vi "Teleop.vi"(10 "Match Info":T1={"Autonomous Elapsed Seconds"=0.0, "TeleOp Elapsed Seconds"=0.0, "Disabled Elapsed Seconds"=0.0, "Visited Autonomous"=FALSE, "Visited TeleOp"=FALSE, "Visited Disabled"=FALSE, "Autonomous Settings"={"Autonomous Style"=enum."Independent", "VI Refnum"=refnum}}, 11 "Call Context":T2) -> ()   [LabVIEW 2015]
doc: "This VI is called for each TeleOp packet received from the DS where the robot is not disabled. It is often used to read from the joysticks and update I/O or to update setpoints for timed control loops. It should complete and return within 20 milliseconds or it may miss DS packets."
uses:
  <vilib>/Rock Robotics/WPI/DriverStation/WPI_DriverStationDerivedRobotMode.ctl
  <vilib>/Rock Robotics/WPI/DriverStation/WPI_DriverStationMatch Info.ctl
  <vilib>/Rock Robotics/WPI/CAN/TalonSRX/WPI_CANTalonSRX_APIControlMode.ctl
  Global Variables/Temp Variables.vi
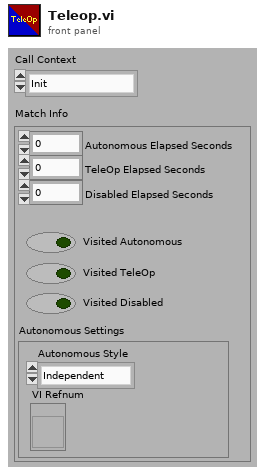
[diagram p1: front panel]
types:
  T1 = typedef "WPI_DriverStationMatch Info.ctl" = cluster{"Autonomous Elapsed Seconds":dbl, "TeleOp Elapsed Seconds":dbl, "Disabled Elapsed Seconds":dbl, "Visited Autonomous":bool, "Visited TeleOp":bool, "Visited Disabled":bool, "Autonomous Settings":cluster{"Autonomous Style":enum16{"Iterative", "Independent"}, "VI Refnum":refnum<vi>}}
  T2 = typedef "WPI_DriverStationDerivedRobotMode.ctl" = enum16{"Init", "Execute", "Stop"}
  T3 = typedef "WPI_CANTalonSRX_APIControlMode.ctl" = enum8{"Percent VBus", "Speed", "Position", "Slave", "Unchanged / Invalid", "Voltage Compensation", "Current", "Motion Profile"}
  T4 = typedef "Robot Control Outputs 2016.ctl" = cluster{"Pilot Left Joystick left-right":dbl, "Pilot Left Joystick up-down":dbl, "Pilot A Button":bool, "Pilot B Button":bool, "Pilot X Button":bool, "Pilot Y Button":bool, "Pilot Left Bumper":bool, "Pilot Right Bumper":bool, "Pilot Back Button":bool, "Pilot Start Button":bool, "Pilot Left Joystick Press":bool, "Pilot Right Joystick Press":bool, "Pilot Left Trigger":dbl, "Pilot Right Joystick left-right":dbl, "Pilot Right Joystick up-down":dbl, "Pilot Right Trigger":dbl, "Copilot Left Joystick left-right":dbl, "Copilot Left Joystick up-down":dbl, "Copilot A Button":bool, "Copilot B Button":bool, "Copilot X Button":bool, "Copilot Y Button":bool, "Copilot Left Bumper":bool, "Copilot Right Bumper":bool, "Copilot Back Button":bool, "Copilot Start Button":bool, "Copilot Left Joystick Press":bool, "Copilot Right Joystick Press":bool, "Copilot Left Trigger":dbl, "Copilot Right Joystick left-right":dbl, "Copilot Right Joystick up-down":dbl, "Copilot Right Trigger":dbl}
  T5 = typedef "Robot Commands 2016.ctl" = cluster{"Robot Forward-Back":dbl, "Robot Twist":dbl, "Fire":bool, "Lift/Drive Shift":bool, "Raise Lifter":bool, "Raise Grabber":bool, "Lower Grabber":bool, "Roller":T6, "Robot Climb Both Sides":dbl, "Grabber to Middle Position":bool, "Grabber to Top Position":bool, "Grabber to Bottom Position":bool, "Robot Climb Left Side":dbl, "Robot Climb Right Side":dbl, "Speed Control Left Side":dbl, "Speed Control Right Side":dbl, "Lower Lifter":bool, "Defense Mode":bool, "Deploy Lifter":bool, "Auto Targetting":bool, "Do the Jiggle":bool}
  T6 = typedef "Roller State.ctl" = enum16{"DONT MOVE", "Intake", "Outtake"}
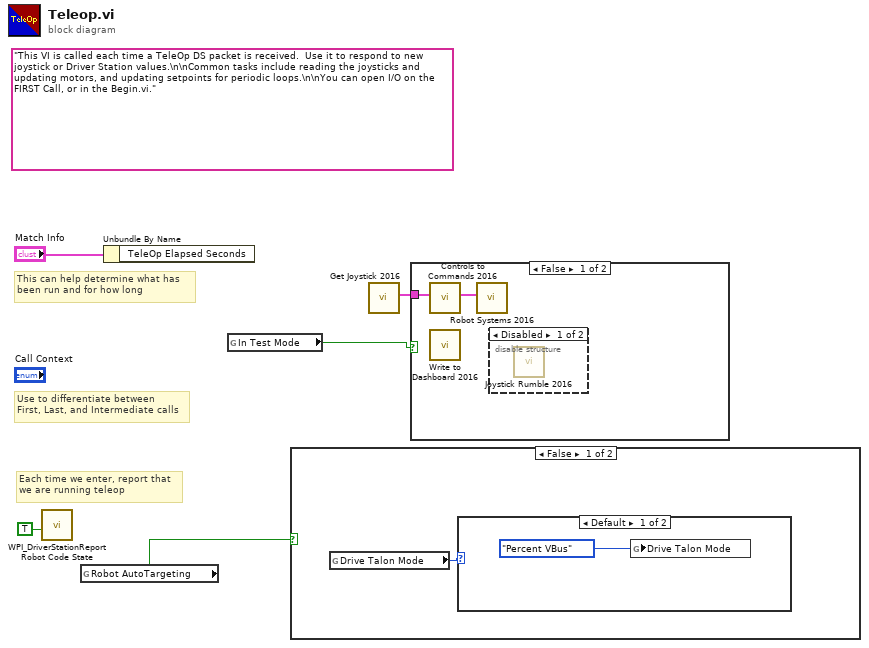
[diagram p0: block diagram]
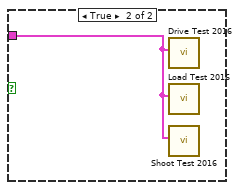
[diagram p5: hidden frame]
diagram:
  (unwired) "This VI is called each time a TeleOp DS packet is received.  Use it to respond to new joystick or Driver Station values.\n\nCommon tasks include reading the joysticks and updating motors, and updating setpoints for periodic loops.\n\nYou can open I/O on the FIRST Call, or in the Begin.vi."
  # "Each time we enter, report that\nwe are running teleop"
  # "Use to differentiate between\nFirst, Last, and Intermediate calls"
  # "This can help determine what has\nbeen run and for how long"
  n1 = call <vilib>:"WPI_DriverStationReport Robot Code State.vi"("TeleOp"=TRUE ("Autonomous")) -> ()  [unwired: 10 in, 1 out]
  n2 = global read "Temp Variables.vi" "Robot AutoTargeting"() -> (w1:bool)
  n3 = Unbundle By Name("Match Info") -> ()  [unwired: 1 out]
  n4 = global read "Temp Variables.vi" "In Test Mode"() -> (w2:bool)
  n5 = case shown="False" w1 {
    frame False {
      n6 = global read "Temp Variables.vi" "Drive Talon Mode"() -> (w6:T3)
      n7 = case shown="Default" w6 {
        frame Default {
          n8 = global write "Temp Variables.vi" "Drive Talon Mode"(WPI_CANTalonSRX_APIControlMode."Percent VBus" ("Drive Talon Mode")) -> ()
        }
        frame "Percent VBus" {
        }
      }
    }
    frame True {
    }
  }
  n9 = call "Get Joystick 2016.vi"() -> ("Pilot-CoPilot Controls"=w3:T4)  [unwired: 11 in]
  n10 = case shown="False" w2 {
    tunnel: w3 -> [w9 w10]
    frame False {
      n11 = call "Controls to Commands 2016.vi"("Pilot-CoPilot Controls"=w9) -> ("Robot Commands"=w8:T5)  [unwired: 10 in]
      n12 = call "Write to Dashboard 2016.vi"() -> ()  [unwired: 12 in]
      n13 = call "Robot Systems 2016.vi"("Robot Commands"=w8) -> ()  [unwired: 11 in]
      n14 = disable-structure shown="Disabled" {
        frame Disabled {
          n15 = call "Joystick Rumble 2016.vi"() -> ()  [unwired: 12 in]
        }
        frame Enabled {
        }
      }
    }
    frame True {
      n16 = call "Drive Test 2016.vi"("Pilot-CoPilot Controls"=w10) -> ()  [unwired: 11 in]
      n17 = call "Load Test 2016.vi"("Pilot-CoPilot Controls"=w10) -> ()  [unwired: 11 in]
      n18 = call "Shoot Test 2016.vi"("Pilot-CoPilot Controls"=w10) -> ()  [unwired: 11 in]
    }
  }
